vi "Lab2_Tick.vi"() -> ()   [LabVIEW 2022 SP3]
uses:
  <vilib>/DAQmx/write.llb/DAQmx Write (Digital 1D Bool NChan 1Samp 1Line).vi
  <vilib>/DAQmx/miscellaneous.llb/DAQmx Fill In Error Info.vi
panel:
  out "Texec [ms]":u32
  in  "Leds Bool":bool[](array[boolean])
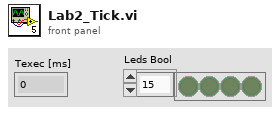
[diagram p1: front panel]
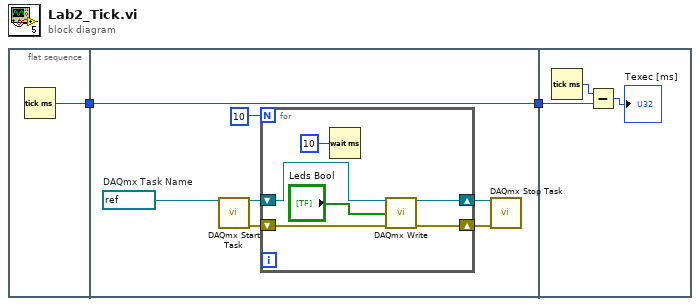
[diagram p0: block diagram]
diagram:
  n1 = flat-sequence {
    tunnel: [w3] -> w1
    tunnel: [w4] -> w2
    tunnel: w1 -> [w4]
    tunnel: w2 -> [w17]
    frame #0 {
      n2 = Tick Count (ms)() -> (millisecond timer value=w3:u32)
    }
    frame #1 {
      w10 = refnum<k21> "LEDs"  # DAQmx Task Name
      n3 = call <vilib>:"DAQmx Start Task.vi"("task/channels in"=w10) -> ("task out"=w9:refnum<k21>, "error out"=w8:errorcluster)  [unwired: 13 in]
      n4 = for {
        N: 10 -> [_]
        shift-right: [w13] -> w7
        shift-left: w9 -> [w15]
        shift-right: [w12] -> w6
        shift-left: w8 -> [w14]
        n5 = Wait (ms)(milliseconds to wait=10) -> ()  [unwired: 1 out]
        n6 = call-poly <vilib>:"DAQmx Write.vi"("task/channels in"=w15, "data"="Leds Bool", "error in"=w14) -> ("task out"=w13:refnum<k21>, "error out"=w12:errorcluster)  [unwired: 10 in, 1 out]
      }
      n7 = call <vilib>:"DAQmx Stop Task.vi"("task/channels in"=w7, "error in"=w6) -> ()  [unwired: 12 in, 2 out]
    }
    frame #2 {
      n8 = Tick Count (ms)() -> (millisecond timer value=w19:u32)
      n9 = Subtract(x=w19, y=w17) -> (x-y=→"Texec [ms]":u32)
    }
  }
